vi "OilValveAmperage.vi"() -> ()   [LabVIEW 2017]
uses:
  <vilib>/eio/EIONode/EIONode.xnode
  <vilib>/rvi/eio/common/nirviEmuTemplateMethod_errors.vi
  <vilib>/eio/EIOPropertyNode/EIOPropertyNode.xnode
  <vilib>/rvi/eio/common/nirviEmuTemplatePropertyGet_errors.vi
  <vilib>/rvi/eio/common/nirviEmuTemplatePropertyGet_noerrors.vi
  <vilib>/rvi/eio/common/nirviEmuTemplatePropertySet_errors.vi
  <vilib>/rvi/eio/common/nirviEmuTemplatePropertySet_noerrors.vi
  <vilib>/rvi/DataTransferAndStorage/Container/XNode/niFpgaContainer.xnode
  <vilib>/rvi/interface/RandomDataEmulation/nirviRandomDataFpgaReadWriteTemplate.vi
  <vilib>/LabVIEW Targets/FPGA/cRIO/shared/nicrio_ModuleControls/nicrio_cRIO-9227_DataRatesRing.ctl
panel:
  out "Data FIFO Full":bool
  in  "Data Rate":T1=1 items=["50.000 kS/s (NI 9227)"=1, "25.000 kS/s (NI 9227)"=2, "16.667 kS/s (NI 9227)"=3, "12.500 kS/s (NI 9227)"=4, "10.000 kS/s (NI 9227)"=5, "8.333 kS/s (NI 9227)"=6, "7.143 kS/s (NI 9227)"=7, "6.250 kS/s (NI 9227)"=8, "5.556 kS/s (NI 9227)"=9, "5.000 kS/s (NI 9227)"=10, "4.545 kS/s (NI 9227)"=11, "4.167 kS/s (NI 9227)"=12, "3.846 kS/s (NI 9227)"=13, "3.571 kS/s (NI 9227)"=14, "3.333 kS/s (NI 9227)"=15, "3.125 kS/s (NI 9227)"=16, "2.941 kS/s (NI 9227)"=17, "2.778 kS/s (NI 9227)"=18, "2.632 kS/s (NI 9227)"=19, "2.500 kS/s (NI 9227)"=20, "2.381 kS/s (NI 9227)"=21, "2.273 kS/s (NI 9227)"=22, "2.174 kS/s (NI 9227)"=23, "2.083 kS/s (NI 9227)"=24, "2.000 kS/s (NI 9227)"=25, "1.923 kS/s (NI 9227)"=26, "1.852 kS/s (NI 9227)"=27, "1.786 kS/s (NI 9227)"=28, "1.724 kS/s (NI 9227)"=29, "1.667 kS/s (NI 9227)"=30, "1.613 kS/s (NI 9227)"=31]
  out "FPGA Error Out":errorcluster
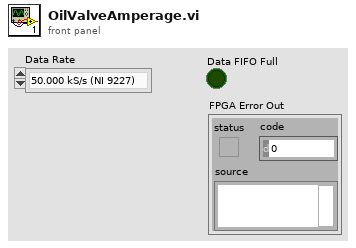
[diagram p1: front panel]
types:
  T1 = typedef "nicrio_cRIO-9227_DataRatesRing.ctl" = u8
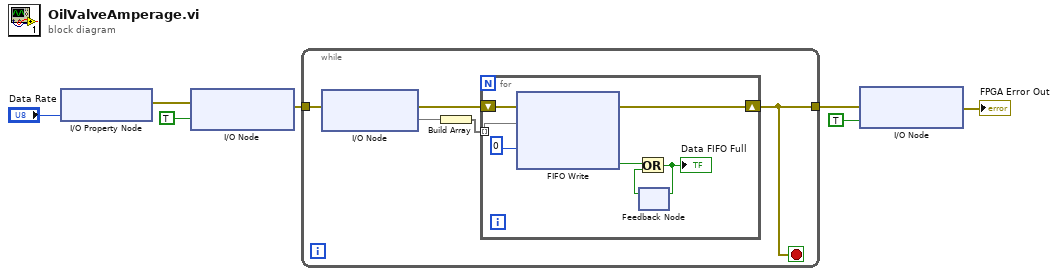
[diagram p0: block diagram]
diagram:
  n1 = xnode "I/O Property Node"("Data Rate"="Data Rate") -> ("error out"=w7:errorcluster)  [unwired: 2 in, 1 out]
  n2 = xnode "I/O Node"("error in"=w7, "Mod1/Start"=TRUE) -> ("error out"=w3:errorcluster)  [unwired: 1 in, 1 out]
  n3 = while {
    tunnel: [w11] -> w5
    tunnel: w3 -> [w12]
    stop <- w11 stop-if-true
    n4 = xnode "I/O Node"("error in"=w12) -> ("error out"=w8:errorcluster, "Mod1/AI0"=w10)  [unwired: 1 in, 1 out]
    n5 = Build Array(w10) -> (w9:void[])
    n6 = for {
      tunnel: w9 -> [w15] mode=indexing
      shift-right: [w13] -> w11
      shift-left: w8 -> [w14]
      n7 = xnode ("FIFO Write")("Element"=w15, "Timeout"=0 ("Timeout (-1 for no timeout)"), "error in (no error)"=w14) -> ("Timed Out?"=w17:bool, "error out"=w13:errorcluster)  [unwired: 1 in, 1 out]
      n8 = feedback #1() -> (w19:bool)  [unwired: 1 out]
      n9 = Or(x=w17, y=w19) -> (x .or. y?=w18:bool)
      "Data FIFO Full" <- w18
      n10 = feedback-in #1(w18) -> ()
    }
  }
  n11 = xnode "I/O Node"("error in"=w5, "Mod1/Stop"=TRUE) -> ("error out"=→"FPGA Error Out":errorcluster)  [unwired: 1 in, 1 out]
